vi "globalVariables.vi"() -> ()   [LabVIEW 2021]
panel:
  in  "dataLogPath":path
  in  "syringeTotalVol":dbl
  in  "Motion":T1={"Top Speed (5000 sps) "=3000, "Start Speed (750 sps)"=750, "Stop Speed (750 sps)"=750, "Accel (17500 st/s^2)"=17500, "Decel (17500 st/s^2)"=17500, "Backlash Steps (100 steps)"=100}
  in  "cDAQDirection_p2":tag="cDAQ1Mod1/port0/line1"
  in  "cDAQVoltage_p2":tag="cDAQ1Mod2/ao1"
  in  "cDAQDirection_p1":tag="cDAQ1Mod1/port0/line0"
  in  "cDAQVoltage_p1":tag="cDAQ1Mod2/ao0"
  in  "robotName":string="a1"
  in  "pumpReverseVol":dbl
  in  "syringeReverseVol":dbl
  out "valvePosition":dbl
  out "syringePosition":dbl
  out "syringeBusy":bool
  in  "rate_p2":dbl caption="rate_p1" format="%#_2g"
  in  "rate_p1":dbl format="%#_2g"
  in  "voltage_p2":dbl
  in  "time_p2":dbl
  in  "voltage_p1":dbl
  in  "time_p1":dbl
  # "STAR System"
  # "Syringe"
  # "Pumps"
  # "cDAQ"
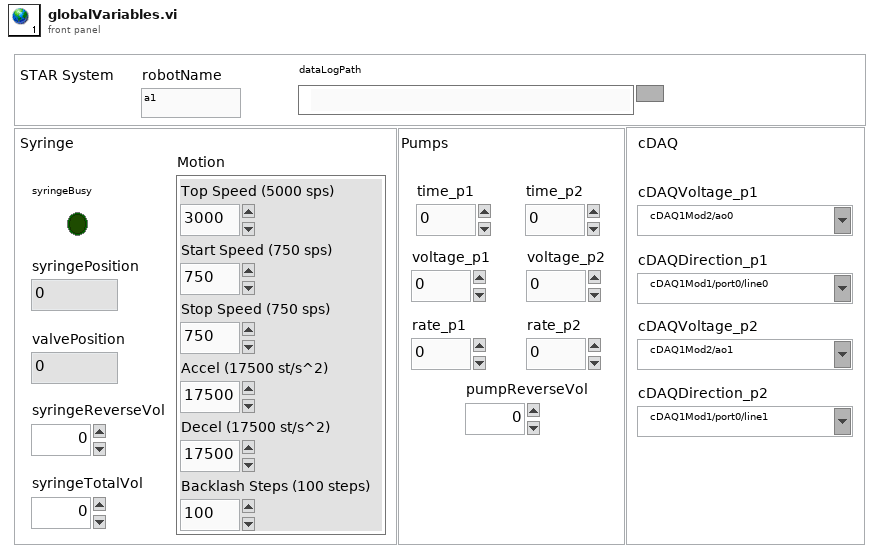
[diagram p1: front panel]
types:
  T1 = cluster{"Top Speed (5000 sps) ":i32, "Start Speed (750 sps)":i32, "Stop Speed (750 sps)":i32, "Accel (17500 st/s^2)":i32, "Decel (17500 st/s^2)":i32, "Backlash Steps (100 steps)":i32}
diagram:
